vi "Get Pos Data.vi"(11 "AttMap":map{string, string}(c390)) -> (3 "Position":T1)   [LabVIEW 2025]
uses:
  <vilib>/Utility/miscctls.llb/LVPointTypeDef.ctl
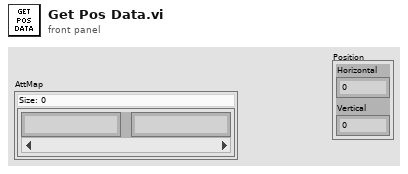
[diagram p1: front panel]
types:
  T1 = typedef "LVPointTypeDef.ctl" = cluster{"Horizontal":i16, "Vertical":i16}
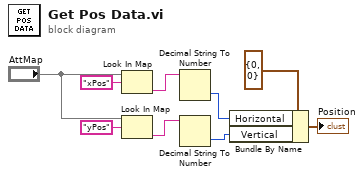
[diagram p0: block diagram]
diagram:
  n1 = Look In Map(map="AttMap", key="xPos") -> (value=w5:string)  [unwired: 1 in, 1 out]
  n2 = Look In Map(map="AttMap", key="yPos") -> (value=w6:string)  [unwired: 1 in, 1 out]
  n3 = Decimal String To Number(string=w5) -> (number=w8:i32)  [unwired: 2 in, 1 out]
  n4 = Decimal String To Number(string=w6) -> (number=w9:i32)  [unwired: 2 in, 1 out]
  n5 = Bundle By Name(cluster=T1 {"Horizontal"=0, "Vertical"=0} ("location"), "Horizontal"=w8, "Vertical"=w9) -> (→"Position":T1)
